vi "Arm Start Trigger 2012 NIVerified.vi"() -> ()   [LabVIEW 2012]
doc: "I. Description:\nThis example demonstrates how to count digital events on a Counter Input Channel. The Initial Count, Count Direction, and Edge are all configurable. \n\nEdges are counted on the counter's default input terminal (refer to section IV, I/O Connections Overview, below for more information), but could easily be modified to count edges on a PFI or RTSI line.\n\nII. Instructions for Running:\n1. Select the Physical Channel which corresponds to the counter you want to count edges on the DAQ device.\n2. Enter the Initial Count, Count Direction, and measurement Edge to specify how you want the counter to count. Additionally, you can change the input terminal where events are counted using the channel property node.\nNote: Use the Gen Dig Pulse Train-Continuous example to verify that you are counting correctly on the DAQ device.\n\nIII. Block Diagram Steps:\n1. Create a Counter Input channel to Count Events. The Edge parameter is used to determine if the counter will increment on rising or falling edges.\n2. Call the Start VI to arm the counter and begin counting. The counter will be preloaded with the Initial Count.\n3. The counter will be continually polled until the Stop button is pressed on the front panel.\n4. Call the Clear Task VI to clear the Task.\n5. Use the popup dialog box to display an error if any.\n\nIV. I/O Connections Overview:\nThe counter will count edges on the input terminal of the counter specified in the Physical Channel I/O control.\n\nIn this example the counter will count edges on the default input terminal on ctr0.\n\nFor more information on the default counter input and output terminals for your device, open the NI-DAQmx Help, and refer to Counter Signal Connections found under the Device Considerations book in the table of contents."
uses:
  <vilib>/Utility/error.llb/DialogType.ctl
  <vilib>/DAQmx/configure/timing.llb/DAQmx Timing (Sample Clock).vi
  <vilib>/DAQmx/create/channels.llb/DAQmx Create Channel (CI-Count Edges).vi
  <vilib>/DAQmx/configure/timing.llb/DAQmx Timing (Implicit).vi
  <vilib>/DAQmx/create/channels.llb/DAQmx Create Channel (CO-Pulse Generation-Frequency).vi
  <vilib>/DAQmx/read.llb/DAQmx Read (Counter 1D DBL 1Chan NSamp).vi
  <resource>/objmgr/daqmx.rc
panel:
  in  "Number of Samples CTR1":i32=1000
  in  "Number os Samples CTR0":i32=1000
  out "data 2":dbl[](array[numeric]) caption="Counter 1 Data" format="%0.2f"
  out "data":dbl[](array[numeric]) caption="Counter 0 Data" format="%0.2f"
  in  "Arm Start Source":tag="/Dev5/PFI0"
  in  "Counter(s) 2":tag="Dev5/ctr1" caption="Counter 1"
  in  "Initial Count 2":u32 caption="Initial Count"
  in  "Count Direction 2":i32(ring)=10128 caption="Count Direction" items=["Count Up"=10128, "Count Down"=10124, "Externally Controlled"=10326]
  in  "Edge 2":i32(ring)=10280 caption="Edge" items=["Rising"=10280, "Falling"=10171]
  in  "Edge":i32(ring)=10280 items=["Rising"=10280, "Falling"=10171]
  in  "Count Direction":i32(ring)=10128 items=["Count Up"=10128, "Count Down"=10124, "Externally Controlled"=10326]
  in  "Initial Count":u32
  in  "Counter(s)":tag="Dev5/ctr0" caption="Counter 0"
  in  "stop":bool
  # "Overview:The VI is used an Arm Start Trigger for both counters. The Arm Start Trigger is set using a DAQmx Trigger Property node.\nRequirements: \n•\tLabVIEW 2012 (or compatible)\n•\tNI DAQmx 12.0 (or compatible)\nInstructions:\n1. Select the Physical Channel which corresponds to the counter you want to count edges on the DAQ device.\n2.  Enter the Initial Count, Count Direction, and measurement Edge to specify how you want the counter to count.  Additionally, you can change the input terminal where events are counted using the channel property node.\n3. Run the VI."
  # "Channel Parameters"
  # "Channel Parameters"
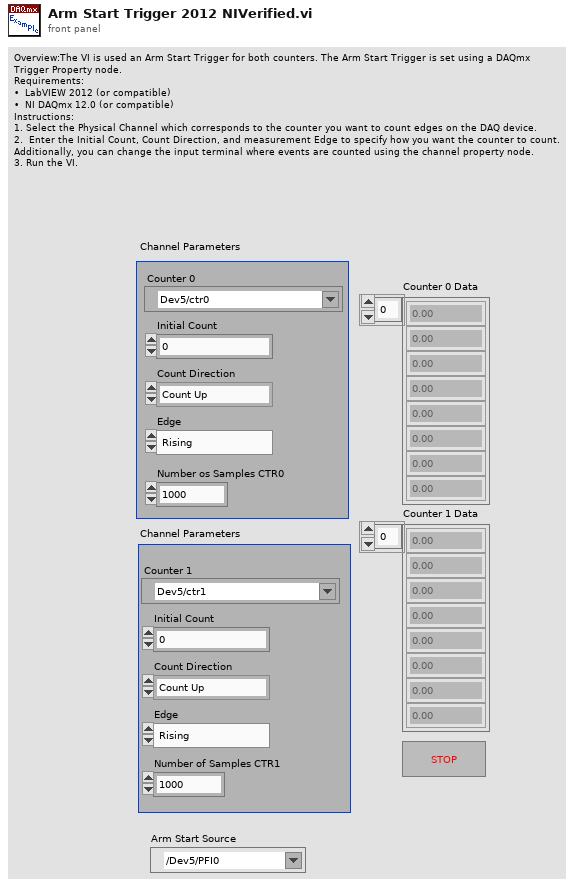
[diagram p1: front panel]
types:
  T1 = typedef "DialogType.ctl" = u16
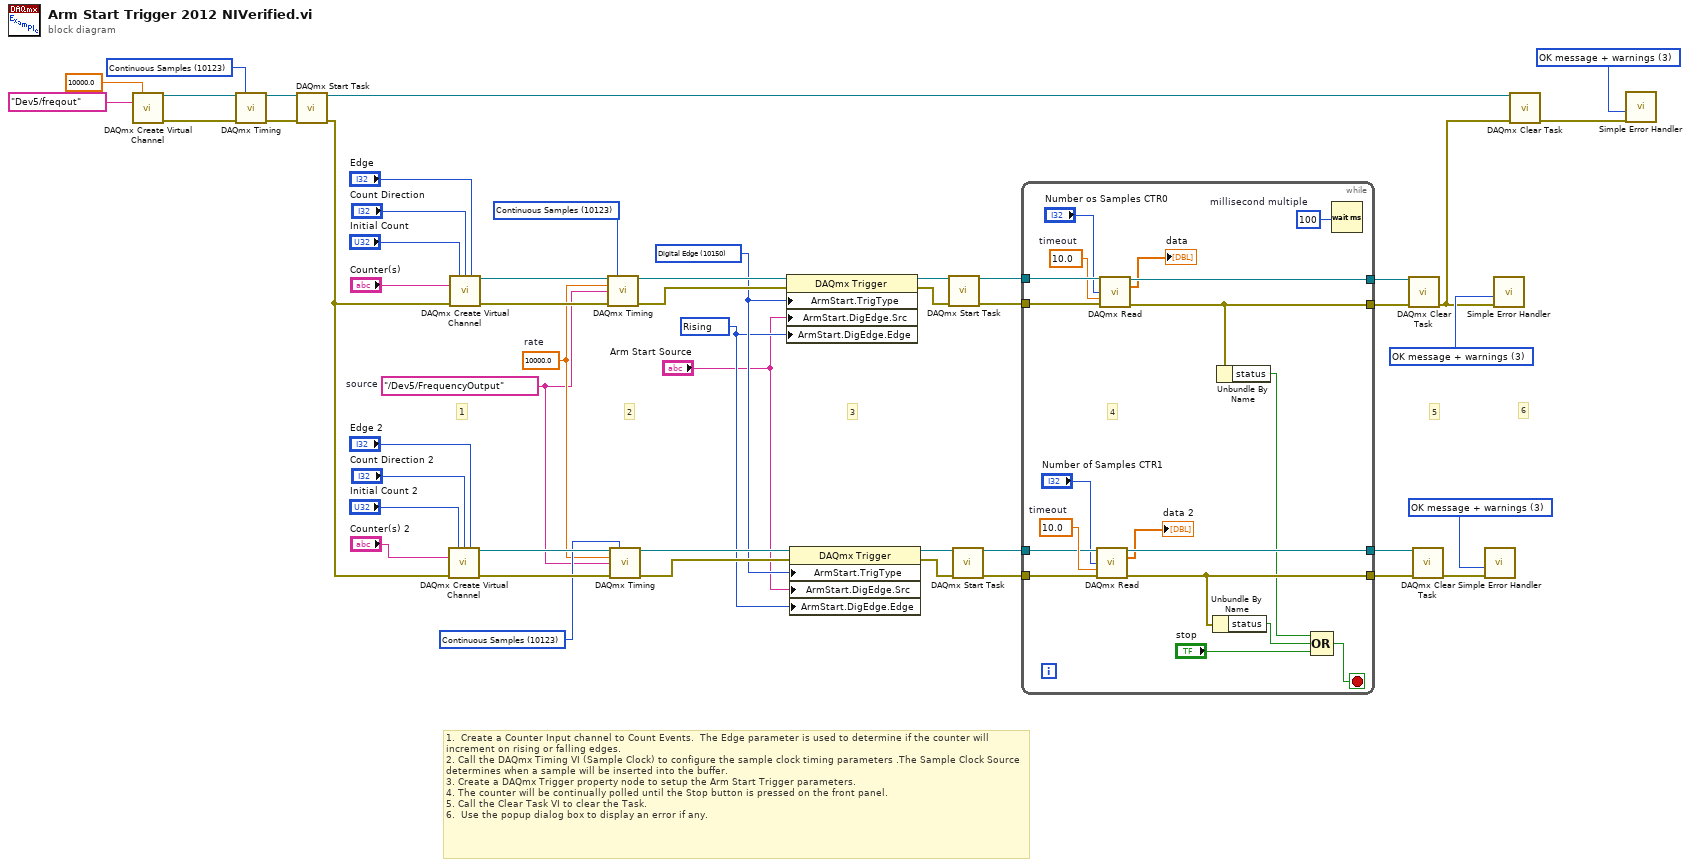
[diagram p0: block diagram]
diagram:
  w1 = T1 3 items=["no dialog", "OK message", "continue or stop message", "OK message + warnings", "continue/stop + warnings"] ("type of dialog (OK msg:1)")
  w8 = 10123 items=["Finite Samples"=10178, "Continuous Samples"=10123, "Hardware Timed Single Point"=12522] ("sample mode")
  w18 = 10123 items=["Finite Samples"=10178, "Continuous Samples"=10123, "Hardware Timed Single Point"=12522] ("sample mode")
  w19 = 10123 items=["Finite Samples"=10178, "Continuous Samples"=10123, "Hardware Timed Single Point"=12522] ("sample mode")
  w14 = 10000.0  # rate
  w13 = tag "/Dev5/FrequencyOutput"  # source
  w16 = 10280 items=["Rising"=10280, "Falling"=10171] ("ArmStart.DigEdge.Edge")
  w17 = 10150 items=["Digital Edge"=10150, "None"=10230] ("ArmStart.TrigType")
  w39 = T1 3 items=["no dialog", "OK message", "continue or stop message", "OK message + warnings", "continue/stop + warnings"] ("type of dialog (OK msg:1)")
  w42 = T1 3 items=["no dialog", "OK message", "continue or stop message", "OK message + warnings", "continue/stop + warnings"] ("type of dialog (OK msg:1)")
  # "6"
  # "1.  Create a Counter Input channel to Count Events.  The Edge parameter is used to determine if the counter will increment on rising or falling edges.\n2. Call the DAQmx Timing VI (Sample Clock) to configure the sample clock timing parameters .The Sample Clock Source determines when a sample will be inserted into the buffer.\n3. Create a DAQmx Trigger property node to setup the Arm Start Trigger parameters.\n4. The counter will be continually polled until the Stop button is pressed on the front panel.\n5. Call the Clear Task VI to clear the Task.\n6.  Use the popup dialog box to display an error if any."
  # "5"
  # "3"
  # "2"
  # "1"
  n1 = call-poly <vilib>:"DAQmx Create Virtual Channel.vi"("frequency"=10000.0, "counter"=tag "Dev5/freqout" ("physical channels")) -> ("task out"=w12:refnum<k21>, "error out"=w10:errorcluster)  [unwired: 7 in, 5 out]
  n2 = call-poly <vilib>:"DAQmx Timing.vi"("task/channels in"=w12, "sample mode"=w8, "error in"=w10) -> ("task out"=w11:refnum<k21>, "error out"=w9:errorcluster)  [unwired: 1 in, 10 out]
  n3 = call <vilib>:"DAQmx Start Task.vi"("task/channels in"=w11, "error in"=w9) -> ("task out"=w4:refnum<k21>, "error out"=w6:errorcluster)  [unwired: 12 out]
  n4 = call-poly <vilib>:"DAQmx Create Virtual Channel.vi"("initial count"="Initial Count 2", "count direction"="Count Direction 2", "edge"="Edge 2", "counter"="Counter(s) 2", "error in"=w6) -> ("task out"=w30:refnum<k21>, "error out"=w31:errorcluster)  [unwired: 2 in, 7 out]
  n5 = call-poly <vilib>:"DAQmx Create Virtual Channel.vi"("initial count"="Initial Count", "count direction"="Count Direction", "edge"="Edge", "counter"="Counter(s)", "error in"=w6) -> ("task out"=w37:refnum<k21>, "error out"=w36:errorcluster)  [unwired: 2 in, 7 out]
  n6 = call-poly <vilib>:"DAQmx Timing.vi"("task/channels in"=w37, "sample mode"=w19, "rate"=w14, "source"=w13, "error in"=w36) -> ("task out"=w35:refnum<k21>, "error out"=w34:errorcluster)  [unwired: 2 in, 7 out]
  n7 = call-poly <vilib>:"DAQmx Timing.vi"("task/channels in"=w30, "sample mode"=w18, "rate"=w14, "source"=w13, "error in"=w31) -> ("task out"=w32:refnum<k21>, "error out"=w33:errorcluster)  [unwired: 2 in, 7 out]
  n8 = property class="DAQmx Trigger"(reference=w35, error in=w34, "ArmStart.TrigType"=w17, "ArmStart.DigEdge.Src"="Arm Start Source", "ArmStart.DigEdge.Edge"=w16) -> (reference out=w41:refnum<k21>, error out=w40:errorcluster)
  n9 = property class="DAQmx Trigger"(reference=w32, error in=w33, "ArmStart.TrigType"=w17, "ArmStart.DigEdge.Src"="Arm Start Source", "ArmStart.DigEdge.Edge"=w16) -> (reference out=w25:refnum<k21>, error out=w24:errorcluster)
  n10 = call <vilib>:"DAQmx Start Task.vi"("task/channels in"=w41, "error in"=w40) -> ("task out"=w48:refnum<k21>, "error out"=w50:errorcluster)  [unwired: 12 out]
  n11 = call <vilib>:"DAQmx Start Task.vi"("task/channels in"=w25, "error in"=w24) -> ("task out"=w23:refnum<k21>, "error out"=w22:errorcluster)  [unwired: 12 out]
  n12 = while {
    tunnel: w50 -> [w69]
    tunnel: [w65] -> w49
    tunnel: w48 -> [w68]
    tunnel: [w67] -> w47
    tunnel: w23 -> [w63]
    tunnel: w22 -> [w62]
    tunnel: [w61] -> w21
    tunnel: [w60] -> w20
    stop <- w56 stop-if-true
    w64 = 10.0  # timeout
    w51 = u32 100  # millisecond multiple
    w66 = 10.0  # timeout
    # "4"
    n13 = call-poly <vilib>:"DAQmx Read.vi"("task/channels in"=w63, "number of samples per channel"="Number of Samples CTR1", "timeout"=w64, "error in"=w62) -> ("task out"=w61:refnum<k21>, "data"=→"data 2":dbl[], "error out"=w60:errorcluster)  [unwired: 9 out]
    n14 = call-poly <vilib>:"DAQmx Read.vi"("task/channels in"=w68, "number of samples per channel"="Number os Samples CTR0", "timeout"=w66, "error in"=w69) -> ("task out"=w67:refnum<k21>, "data"=→"data":dbl[], "error out"=w65:errorcluster)  [unwired: 9 out]
    n15 = Unbundle By Name(w60) -> ("status"=w58:bool)
    n16 = Unbundle By Name(w65) -> ("status"=w59:bool)
    n17 = Compound Arithmetic op=OR(w59, w58, "stop") -> (w56:bool)
    n18 = Wait (ms)(milliseconds to wait=w51) -> ()  [unwired: 1 out]
  }
  n19 = call <vilib>:"DAQmx Clear Task.vi"("task in"=w47, "error in"=w49) -> ("error out"=w5:errorcluster)  [unwired: 13 out]
  n20 = call <vilib>:"DAQmx Clear Task.vi"("task in"=w21, "error in"=w20) -> ("error out"=w38:errorcluster)  [unwired: 13 out]
  n21 = call <vilib>:"Simple Error Handler.vi"("type of dialog (OK msg:1)"=w39, "error in (no error)"=w38) -> ()  [unwired: 8 out]
  n22 = call <vilib>:"Simple Error Handler.vi"("type of dialog (OK msg:1)"=w42, "error in (no error)"=w5) -> ()  [unwired: 8 out]
  n23 = call <vilib>:"DAQmx Clear Task.vi"("task in"=w4, "error in"=w5) -> ("error out"=w2:errorcluster)  [unwired: 13 out]
  n24 = call <vilib>:"Simple Error Handler.vi"("type of dialog (OK msg:1)"=w1, "error in (no error)"=w2) -> ()  [unwired: 8 out]
